vi "setcoefficientjob.vi"(0 "sample port":refnum<visa-resource-name>[](array[refnum]), 2 "sample sn":string[](array[string])) -> (7 "Array":bool[](array[boolean]))   [LabVIEW 2012]
uses:
  <vilib>/Analysis/Matrix/Datatypes/RealMatrix.ctl
  globalstatus.vi
  globalreport.vi
  globalsettings.vi
  <vilib>/Analysis/Matrix/NI_Matrix.lvlib
panel:
  out "A":T1
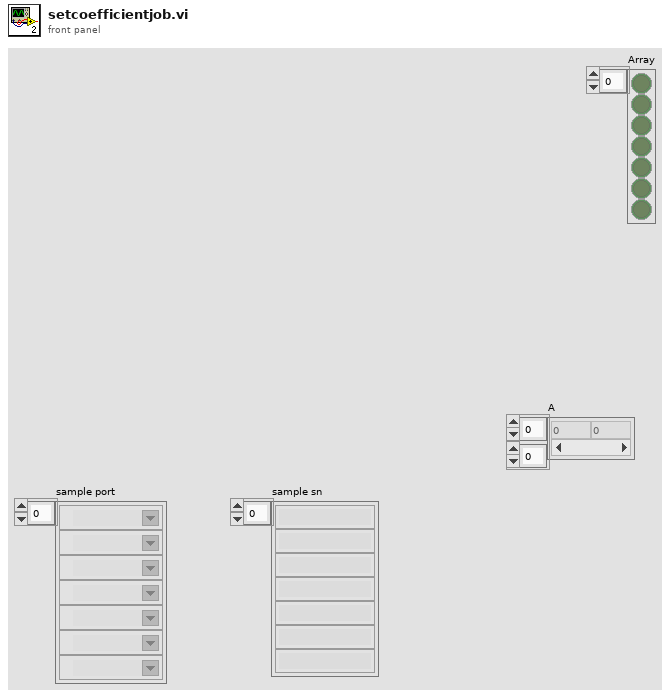
[diagram p1: front panel]
types:
  T1 = typedef "NI_Matrix.lvlib/RealMatrix.ctl" = dbl[][]
  T2 = cluster{"PORT":string, "SN":string, "RED DAC":dbl, "BLUE DAC":dbl, "RED AMP":dbl, "BLUE AMP":dbl, "T0":dbl, "T1":dbl, "T2":dbl, "T3":dbl, "T4":dbl, "T5":dbl, "T6":dbl, "A0":dbl, "A1":dbl, "A2":dbl, "A3":dbl, "B0":dbl, "B1":dbl, "B2":dbl, "C1":dbl, "C0":dbl, "result":string, "error":string}[]
  T3 = cluster{"PORT":string, "SN":string, "RED DAC":dbl, "BLUE DAC":dbl, "RED AMP":dbl, "BLUE AMP":dbl, "Numeric":dbl, "Numeric":dbl, "Numeric":dbl, "Numeric":dbl, "Numeric":dbl, "Numeric":dbl, "Numeric":dbl, dbl, dbl, dbl, dbl, "B0":dbl, "B1":dbl, "B2":dbl, "C1":dbl, "C0":dbl, "result":string, "error":string}
  T4 = cluster{"B0":dbl, "B1":dbl, "K":dbl, "B":dbl, "B2":dbl}
  T5 = cluster{"PORT":string, "SN":string, "RED DAC":dbl, "BLUE DAC":dbl, "RED AMP":dbl, "BLUE AMP":dbl, "T0":dbl, "T1":dbl, "T2":dbl, "T3":dbl, "T4":dbl, "T5":dbl, "T6":dbl, "Real Matrix Element":dbl, "Real Matrix Element":dbl, "Real Matrix Element":dbl, "Real Matrix Element":dbl, "B0":dbl, "B1":dbl, "B2":dbl, "B":dbl, "K":dbl, "result":string, "error":string}
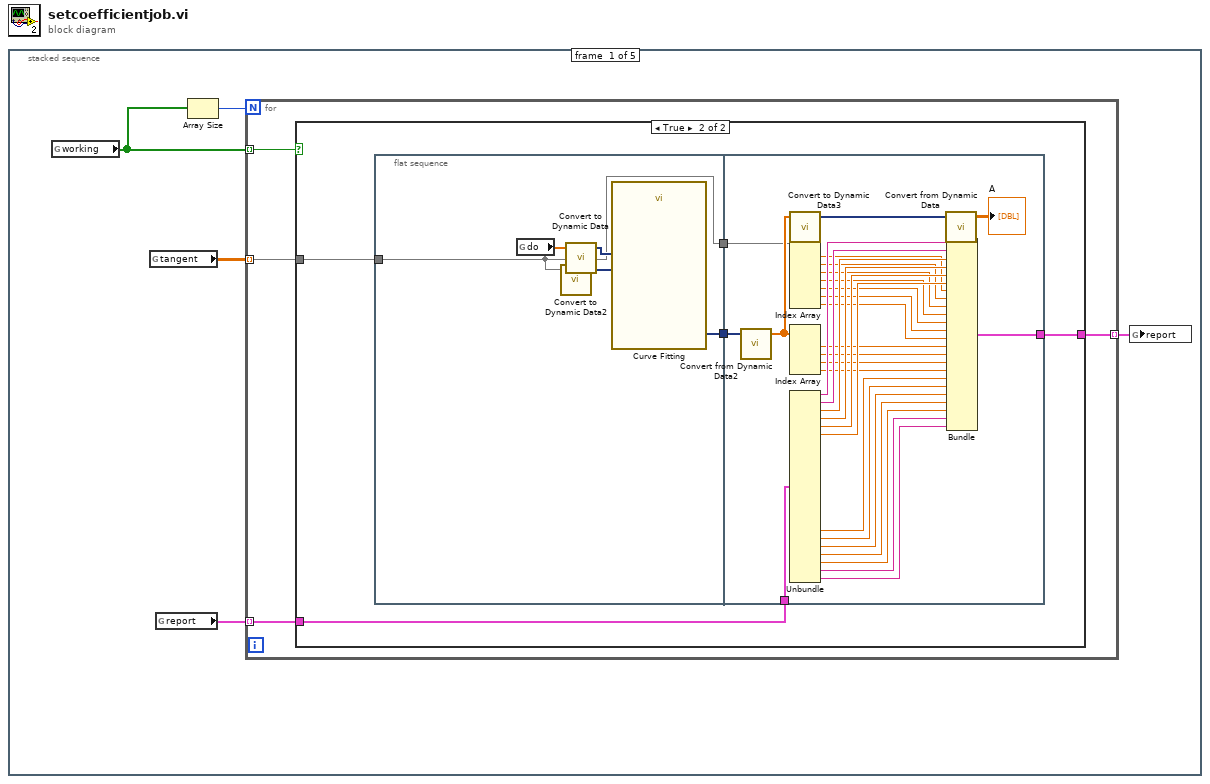
[diagram p0: block diagram]
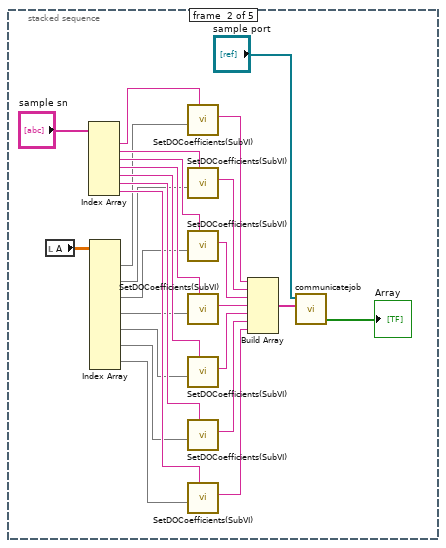
[diagram p3: hidden frame]
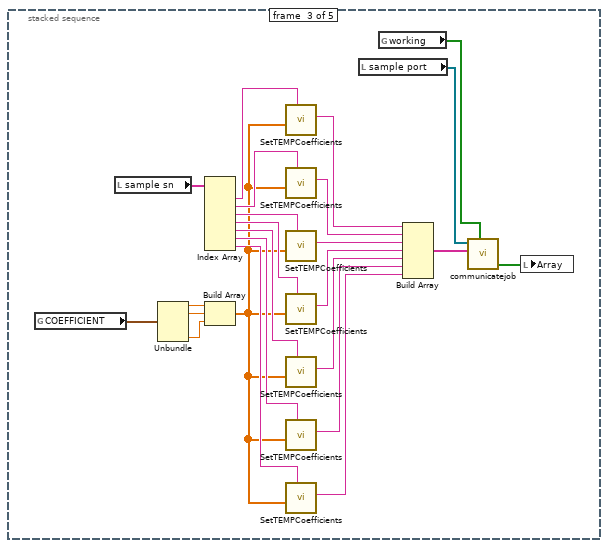
[diagram p4: hidden frame]
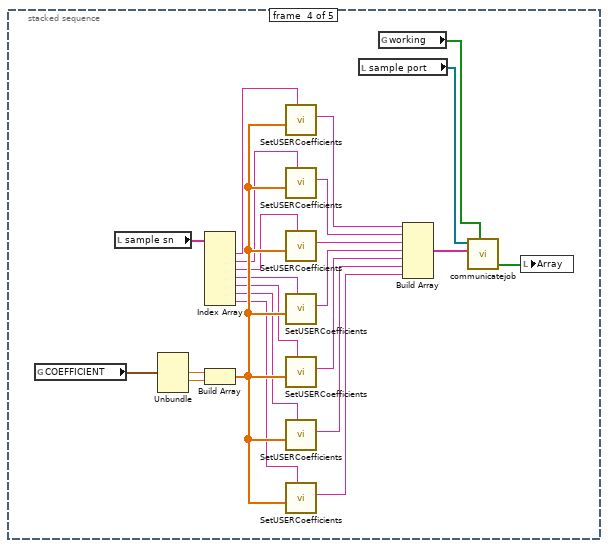
[diagram p5: hidden frame]
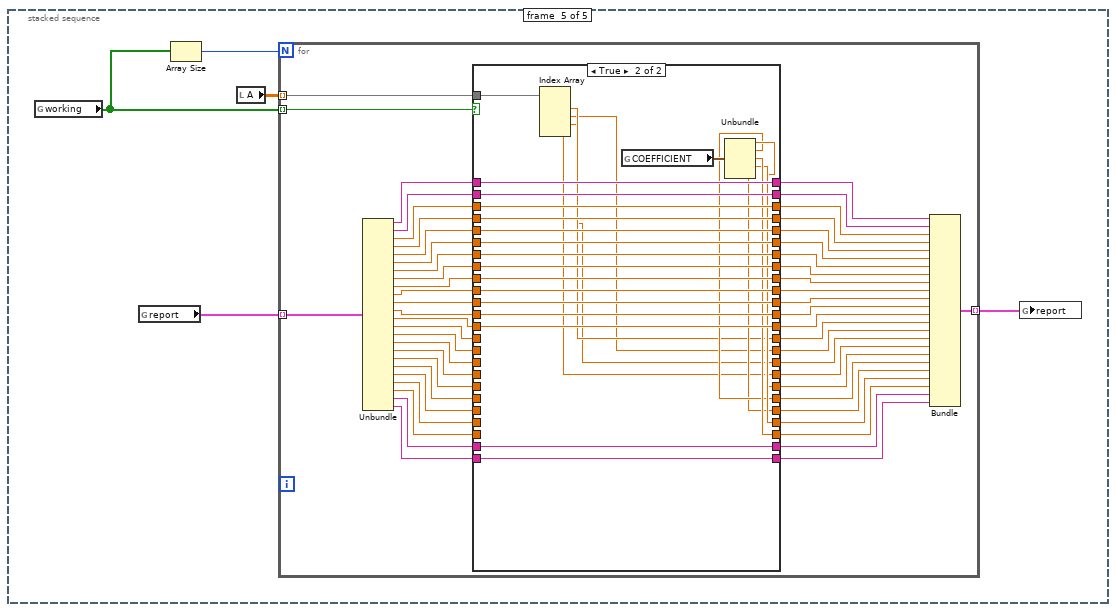
[diagram p6: hidden frame]
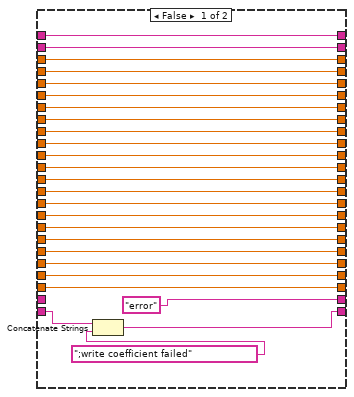
[diagram p7: hidden frame]
diagram:
  n1 = stacked-sequence {
    frame #0 {
      n2 = global read "globalstatus.vi" "working"() -> (w4:bool[])
      n3 = global read "globalstatus.vi" "tangent"() -> (w1:dbl[][])
      n4 = global read "globalreport.vi" "report"() -> (w3:T2)
      n5 = Array Size(array=w4) -> (size(s)=w5:i32)
      n6 = for {
        N: w5 -> [_]
        tunnel: w4 -> [w9] mode=indexing
        tunnel: w1 -> [w8] mode=indexing
        tunnel: w3 -> [w7] mode=indexing
        tunnel: [w6] -> w2 mode=indexing
        n7 = case shown="True" w9 {
          tunnel: w8 -> [_ w15]
          tunnel: w7 -> [w10 w13]
          tunnel: [w10 w11] -> w6
          frame False {
          }
          frame True {
            n8 = flat-sequence {
              tunnel: w15 -> [w16]
              tunnel: [w17] -> w14
              tunnel: [w16] -> w12
              tunnel: w14 -> [w48]
              tunnel: w13 -> [w50]
              tunnel: [w49] -> w11
              tunnel: w12 -> [w45]
              frame #0 {
                n9 = global read "globalstatus.vi" "do"() -> (w20:dbl[])
                n10 = call "Convert to Dynamic Data2"("Array"=w16) -> ("Dynamic Data Type"=w18:dynamicdata)  [unwired: 3 in]
                n11 = call "Convert to Dynamic Data"("Array"=w20) -> ("Dynamic Data Type"=w19:dynamicdata)  [unwired: 3 in]
                n12 = call "Curve Fitting"("Locations"=w18, "Signals"=w19) -> ("polynomial coefficients"=w17:dynamicdata)  [unwired: 5 in, 4 out]
              }
              frame #1 {
                n13 = call "Convert from Dynamic Data2"("Dynamic Data Type"=w48) -> ("Array"=w47:dbl[])  [unwired: 3 in]
                n14 = call "Convert to Dynamic Data3"("Array"=w47) -> ("Dynamic Data Type"=w46:dynamicdata)  [unwired: 3 in]
                n15 = Index Array(array=w45) -> (element #1=w27:dbl, element #2=w26:dbl, element #3=w25:dbl, element #4=w24:dbl, element #5=w23:dbl, element #6=w22:dbl, element #7=w21:dbl)  [unwired: 7 in]
                n16 = Index Array(array=w47) -> (element #1=w31:dbl, element #2=w30:dbl, element #3=w29:dbl, element #4=w28:dbl)  [unwired: 4 in]
                n17 = Unbundle(w50) -> ("PORT"=w44:string, "SN"=w43:string, "RED DAC"=w42:dbl, "BLUE DAC"=w41:dbl, "RED AMP"=w40:dbl, "BLUE AMP"=w39:dbl, "B0"=w38:dbl, "B1"=w37:dbl, "B2"=w36:dbl, "C1"=w35:dbl, "C0"=w34:dbl, "result"=w33:string, "error"=w32:string)  [unwired: 11 out]
                n18 = call "Convert from Dynamic Data"("Dynamic Data Type"=w46) -> ("Array"=→"A":dbl[][])  [unwired: 3 in]
                n19 = Bundle("PORT"=w44, "SN"=w43, "RED DAC"=w42, "BLUE DAC"=w41, "RED AMP"=w40, "BLUE AMP"=w39, "Numeric"=w27, "Numeric"=w26, "Numeric"=w25, "Numeric"=w24, "Numeric"=w23, "Numeric"=w22, "Numeric"=w21, w31, w30, w29, w28, "B0"=w38, "B1"=w37, "B2"=w36, "C1"=w35, "C0"=w34, "result"=w33, "error"=w32) -> (w49:T3)  [unwired: 1 in]
              }
            }
          }
        }
      }
      n20 = global write "globalreport.vi" "report"(w2) -> ()
    }
    frame #1 {
      n21 = local read "A"() -> (w59:T1)
      n22 = Index Array(array="sample sn") -> (element #1=w76:string, element #2=w75:string, element #3=w74:string, element #4=w73:string, element #5=w72:string, element #6=w71:string, element #7=w70:string)  [unwired: 7 in]
      n23 = Index Array(array=w59) -> (element #1=w58:dbl[], element #2=w57:dbl[], element #3=w56:dbl[], element #4=w55:dbl[], element #5=w54:dbl[], element #6=w53:dbl[], element #7=w52:dbl[])  [unwired: 14 in]
      n24 = call "SetDOCoefficients(SubVI).vi"("sn"=w76, "L"=w58) -> ("output frame"=w68:string)  [unwired: 9 in]
      n25 = call "SetDOCoefficients(SubVI).vi"("sn"=w75, "L"=w57) -> ("output frame"=w67:string)  [unwired: 9 in]
      n26 = call "SetDOCoefficients(SubVI).vi"("sn"=w74, "L"=w56) -> ("output frame"=w66:string)  [unwired: 9 in]
      n27 = call "SetDOCoefficients(SubVI).vi"("sn"=w73, "L"=w55) -> ("output frame"=w65:string)  [unwired: 9 in]
      n28 = call "SetDOCoefficients(SubVI).vi"("sn"=w72, "L"=w54) -> ("output frame"=w64:string)  [unwired: 9 in]
      n29 = call "SetDOCoefficients(SubVI).vi"("sn"=w71, "L"=w53) -> ("output frame"=w63:string)  [unwired: 9 in]
      n30 = call "SetDOCoefficients(SubVI).vi"("sn"=w70, "L"=w52) -> ("output frame"=w62:string)  [unwired: 9 in]
      n31 = Build Array(w68, w67, w66, w65, w64, w63, w62) -> (w61:string[])
      n32 = call "communicatejob.vi"("sample port"="sample port", "send command"=w61) -> ("receive result"=→"Array":bool[])  [unwired: 3 in, 3 out]
    }
    frame #2 {
      n33 = global read "globalsettings.vi" "COEFFICIENT"() -> (w82:T4)
      n34 = local read "sample sn"() -> (w98:string[])
      n35 = Unbundle(w82) -> ("B0"=w81:dbl, "B1"=w80:dbl, "B2"=w79:dbl)  [unwired: 2 out]
      n36 = Index Array(array=w98) -> (element #1=w101:string, element #2=w100:string, element #3=w99:string, element #4=w97:string, element #5=w96:string, element #6=w95:string, element #7=w94:string)  [unwired: 7 in]
      n37 = Build Array(w81, w80, w79) -> (w78:dbl[])
      n38 = call "SetTEMPCoefficients.vi"("sn"=w101, "T"=w78) -> ("output frame"=w93:string)  [unwired: 9 in]
      n39 = call "SetTEMPCoefficients.vi"("sn"=w100, "T"=w78) -> ("output frame"=w92:string)  [unwired: 9 in]
      n40 = call "SetTEMPCoefficients.vi"("sn"=w99, "T"=w78) -> ("output frame"=w91:string)  [unwired: 9 in]
      n41 = call "SetTEMPCoefficients.vi"("sn"=w97, "T"=w78) -> ("output frame"=w90:string)  [unwired: 9 in]
      n42 = call "SetTEMPCoefficients.vi"("sn"=w96, "T"=w78) -> ("output frame"=w89:string)  [unwired: 9 in]
      n43 = call "SetTEMPCoefficients.vi"("sn"=w95, "T"=w78) -> ("output frame"=w88:string)  [unwired: 9 in]
      n44 = call "SetTEMPCoefficients.vi"("sn"=w94, "T"=w78) -> ("output frame"=w87:string)  [unwired: 9 in]
      n45 = local read "sample port"() -> (w85:refnum<visa-resource-name>[])
      n46 = global read "globalstatus.vi" "working"() -> (w84:bool[])
      n47 = Build Array(w93, w92, w91, w90, w89, w88, w87) -> (w86:string[])
      n48 = call "communicatejob.vi"("sample port"=w85, "condition"=w84, "send command"=w86) -> ("receive result"=w83:bool[])  [unwired: 2 in, 3 out]
      n49 = local write "Array"(w83) -> ()
    }
    frame #3 {
      n50 = global read "globalsettings.vi" "COEFFICIENT"() -> (w124:T4)
      n51 = local read "sample sn"() -> (w111:string[])
      n52 = Unbundle(w124) -> ("K"=w123:dbl, "B"=w122:dbl)  [unwired: 3 out]
      n53 = Index Array(array=w111) -> (element #1=w110:string, element #2=w109:string, element #3=w108:string, element #4=w107:string, element #5=w106:string, element #6=w105:string, element #7=w104:string)  [unwired: 7 in]
      n54 = Build Array(w123, w122) -> (w121:dbl[])
      n55 = call "SetUSERCoefficients.vi"("sn"=w110, "U"=w121) -> ("output frame"=w120:string)  [unwired: 9 in]
      n56 = call "SetUSERCoefficients.vi"("sn"=w109, "U"=w121) -> ("output frame"=w119:string)  [unwired: 9 in]
      n57 = call "SetUSERCoefficients.vi"("sn"=w108, "U"=w121) -> ("output frame"=w118:string)  [unwired: 9 in]
      n58 = call "SetUSERCoefficients.vi"("sn"=w107, "U"=w121) -> ("output frame"=w117:string)  [unwired: 9 in]
      n59 = call "SetUSERCoefficients.vi"("sn"=w106, "U"=w121) -> ("output frame"=w116:string)  [unwired: 9 in]
      n60 = call "SetUSERCoefficients.vi"("sn"=w105, "U"=w121) -> ("output frame"=w115:string)  [unwired: 9 in]
      n61 = call "SetUSERCoefficients.vi"("sn"=w104, "U"=w121) -> ("output frame"=w114:string)  [unwired: 9 in]
      n62 = local read "sample port"() -> (w103:refnum<visa-resource-name>[])
      n63 = global read "globalstatus.vi" "working"() -> (w112:bool[])
      n64 = Build Array(w120, w119, w118, w117, w116, w115, w114) -> (w113:string[])
      n65 = call "communicatejob.vi"("sample port"=w103, "condition"=w112, "send command"=w113) -> ("receive result"=w102:bool[])  [unwired: 2 in, 3 out]
      n66 = local write "Array"(w102) -> ()
    }
    frame #4 {
      n67 = global read "globalstatus.vi" "working"() -> (w128:bool[])
      n68 = global read "globalreport.vi" "report"() -> (w127:T2)
      n69 = Array Size(array=w128) -> (size(s)=w129:i32)
      n70 = local read "A"() -> (w125:T1)
      n71 = for {
        N: w129 -> [_]
        tunnel: w128 -> [w181] mode=indexing
        tunnel: w127 -> [w178] mode=indexing
        tunnel: [w179] -> w126 mode=indexing
        tunnel: w125 -> [w180] mode=indexing
        n72 = Unbundle(w178) -> ("PORT"=w176:string, "SN"=w175:string, "RED DAC"=w161:dbl, "BLUE DAC"=w173:dbl, "RED AMP"=w171:dbl, "BLUE AMP"=w170:dbl, "T0"=w169:dbl, "T1"=w168:dbl, "T2"=w167:dbl, "T3"=w166:dbl, "T4"=w165:dbl, "T5"=w164:dbl, "T6"=w163:dbl, "A0"=w162:dbl, "A1"=w157:dbl, "A2"=w156:dbl, "A3"=w155:dbl, "B0"=w154:dbl, "B1"=w153:dbl, "B2"=w152:dbl, "C1"=w151:dbl, "C0"=w150:dbl, "result"=w149:string, "error"=w148:string)
        n73 = case shown="True" w181 {
          tunnel: w180 -> [_ w232]
          tunnel: [w207 w231] -> w177
          tunnel: w176 -> [w207 w231]
          tunnel: w175 -> [w206 w230]
          tunnel: [w206 w230] -> w174
          tunnel: w173 -> [w187 w229]
          tunnel: [w187 w229] -> w172
          tunnel: w171 -> [w188 w227]
          tunnel: w170 -> [w189 w226]
          tunnel: w169 -> [w190 w225]
          tunnel: w168 -> [w191 w224]
          tunnel: w167 -> [w192 w223]
          tunnel: w166 -> [w193 w222]
          tunnel: w165 -> [w194 w221]
          tunnel: w164 -> [w195 w220]
          tunnel: w163 -> [w196 w219]
          tunnel: w162 -> [w197 _]
          tunnel: w161 -> [w186 w228]
          tunnel: [w186 w228] -> w160
          tunnel: [w188 w227] -> w159
          tunnel: [w189 w226] -> w158
          tunnel: [w190 w225] -> w147
          tunnel: [w191 w224] -> w146
          tunnel: [w192 w223] -> w145
          tunnel: [w193 w222] -> w144
          tunnel: [w194 w221] -> w143
          tunnel: [w195 w220] -> w142
          tunnel: [w196 w219] -> w141
          tunnel: [w197 w211] -> w140
          tunnel: w157 -> [w198 _]
          tunnel: w156 -> [w199 _]
          tunnel: w155 -> [w200 _]
          tunnel: w154 -> [w201 _]
          tunnel: [w198 w210] -> w139
          tunnel: [w199 w209] -> w138
          tunnel: [w200 w208] -> w137
          tunnel: [w201 w214] -> w136
          tunnel: w153 -> [w202 _]
          tunnel: w152 -> [w203 _]
          tunnel: w151 -> [w204 _]
          tunnel: [w202 w213] -> w135
          tunnel: [w203 w212] -> w134
          tunnel: [w204 w215] -> w133
          tunnel: w150 -> [w205 _]
          tunnel: [w205 w216] -> w132
          tunnel: w149 -> [_ w218]
          tunnel: w148 -> [w184 w217]
          tunnel: ["error" w218] -> w131
          tunnel: [w183 w217] -> w130
          frame False {
            n74 = Concatenate Strings(w184, ";write coefficient failed") -> (w183:string)
          }
          frame True {
            n75 = Index Array(array=w232) -> (element #1=w211:dbl, element #2=w210:dbl, element #3=w209:dbl, element #4=w208:dbl)  [unwired: 4 in]
            n76 = global read "globalsettings.vi" "COEFFICIENT"() -> (w233:T4)
            n77 = Unbundle(w233) -> ("B0"=w214:dbl, "B1"=w213:dbl, "K"=w216:dbl, "B"=w215:dbl, "B2"=w212:dbl)
          }
        }
        n78 = Bundle("PORT"=w177, "SN"=w174, "RED DAC"=w160, "BLUE DAC"=w172, "RED AMP"=w159, "BLUE AMP"=w158, "T0"=w147, "T1"=w146, "T2"=w145, "T3"=w144, "T4"=w143, "T5"=w142, "T6"=w141, "Real Matrix Element"=w140, "Real Matrix Element"=w139, "Real Matrix Element"=w138, "Real Matrix Element"=w137, "B0"=w136, "B1"=w135, "B2"=w134, "B"=w133, "K"=w132, "result"=w131, "error"=w130) -> (w179:T5)  [unwired: 1 in]
      }
      n79 = global write "globalreport.vi" "report"(w126) -> ()
    }
  }
